vi "Remove ID.vi"(11 "id string":string) -> (1 "appended number":i32, 2 "name":string, 3 "remaining id string":string)   [LabVIEW 2021, in "DSF Core.lvlib" / "Configuration Session.lvclass"]
uses:
  Configuration Session.lvclass
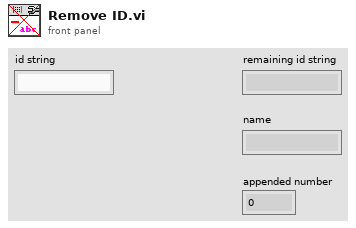
[diagram p1: front panel]
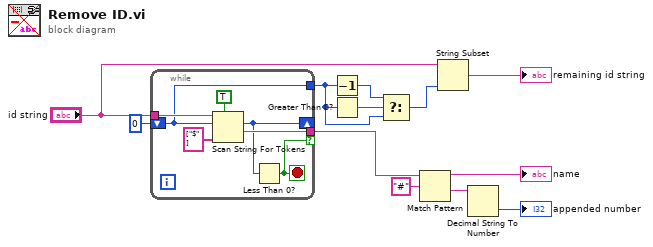
[diagram p0: block diagram]
diagram:
  n1 = while {
    tunnel: "id string" -> [w16]
    tunnel: [w17] -> w4 if=w14
    shift-right: [w15] -> _
    shift-left: 0 ("offset past token") -> [w13]
    tunnel: [w13] -> w8
    stop <- w14 stop-if-true
    n2 = Scan String For Tokens(5:TRUE ("allow empty tokens? (F)"), 6:string[] ["$"] ("delimiters (\\s,\\t,\\r,\\n)"), 8:w13, 9:w16) -> (1:w17:string, 2:w15:i32)  [unwired: 2 in, 2 out]
    n3 = Less Than 0?(x=w15) -> (x < 0?=w14:bool)
  }
  n4 = Decrement(x=w8) -> (x-1=w7:i32)
  n5 = Greater Than 0?(x=w8) -> (x > 0?=w6:bool)
  n6 = Select(t=w7, s=w6, f=w8) -> (s? t:f=w9:i32)
  n7 = Match Pattern(string=w4, regular expression="#") -> (before substring=→"name":string, after substring=w2:string)  [unwired: 1 in, 2 out]
  n8 = String Subset(string="id string", length (rest)=w9) -> (substring=→"remaining id string":string)  [unwired: 1 in]
  n9 = Decimal String To Number(string=w2) -> (number=→"appended number":i32)  [unwired: 2 in, 1 out]
